vi "Find Red Pitayas.vi"(6 "Timeout":i32=100, 7 "Acceptable logic tags":u16[](array[numeric])=[101, 102, 109], 8 "Error In":errorcluster, 9 "End address":i32=120, 10 "Start address":i32=100, 11 "Subnet":string="192.168.1") -> (0 "Error Out":errorcluster, 1 "Addresses":string[](array[string]), 2 "Device names":string[](array[string]), 5 "Logic tags out":u16[](array[numeric])=[101, 102])   [LabVIEW 2019, in "Red Pitaya Digitizer.lvclass"]
uses:
  Red Pitaya Digitizer.lvclass
  RP Core/RP Communicator/RP Communicator.lvclass
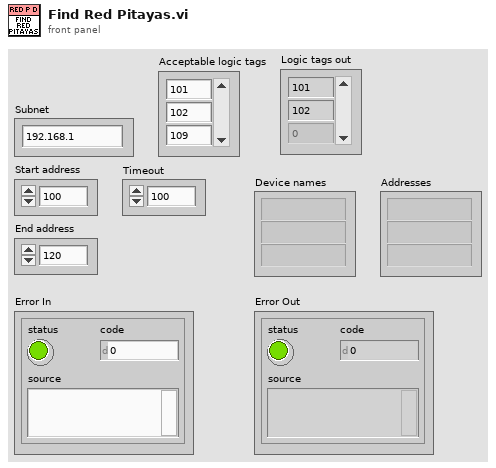
[diagram p1: front panel]
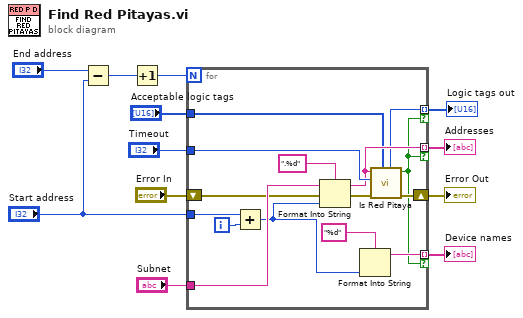
[diagram p0: block diagram]
diagram:
  n1 = Subtract(x="End address", y="Start address") -> (x-y=w11:i32)
  n2 = Increment(x=w11) -> (x+1=w10:i32)
  n3 = for {
    N: w10 -> [_]
    tunnel: "Start address" -> [w25]
    tunnel: "Subnet" -> [w23]
    tunnel: "Timeout" -> [w22]
    tunnel: [w21] -> w5 mode=indexing if=w13
    shift-right: [w19] -> w3
    shift-left: "Error In" -> [w20]
    tunnel: [w16] -> w4 mode=indexing if=w13
    tunnel: "Acceptable logic tags" -> [w15]
    tunnel: [w14] -> w1 mode=indexing if=w13
    i -> [w26]
    n4 = Add(x=w25, y=w26) -> (x+y=w18:i32)
    n5 = Format Into String(format string=".%d", initial string=w23, error in=w20, w18) -> (resulting string=w21:string, error out=w27:errorcluster)
    n6 = Format Into String(format string="%d", w18) -> (resulting string=w16:string)  [unwired: 2 in, 1 out]
    n7 = call "Is Red Pitaya.vi"("Acceptable logic tags"=w15, "Error In"=w27, "Timeout"=w22, "Server address"=w21) -> ("Error Out"=w19:errorcluster, "Red Pitaya"=w13:bool, "Logic tag out"=w14:u16)  [unwired: 3 in, 2 out]
  }
  "Device names" <- w4
  "Error Out" <- w3
  "Addresses" <- w5
  "Logic tags out" <- w1
